vi "MoveBySteps.vi"(0 "Jiaxin_Stepper_Controller in":refnum<class "Jiaxin_Stepper_Controller.lvclass">, 1 "Direction":enum16{"Forward", "Backwards"}(ring)=enum."Backwards", 5 "Steps":dbl, 7 "Channel":u16(ring)=1 items=["Channel1"=1, "Channel2"=2, "Channel3"=3, "Channel4"=4], 9 "Speed":u32, 11 "error in (no error)":errorcluster, 13 "Polarity":enum16{"Positive", "Negative"}(ring)) -> (4 "Jiaxin_Stepper_Controller out":refnum<class "Jiaxin_Stepper_Controller.lvclass">, 15 "error out":errorcluster)   [LabVIEW 2023, in "Jiaxin_Stepper_Controller.lvlib" / "Jiaxin_Stepper_Controller.lvclass"]
uses:
  Jiaxin_Stepper_Controller.lvclass
  Jiaxin_Stepper_Controller.lvclass/Jiaxin_Stepper_Controller.ctl
  Interfaces/AbstractInstrumentClasses/TranslationStages_LV/TranslationStagesComm Messages/StageMoveDone Msg/StageMoveDone Msg.lvclass
  <vilib>/ActorFramework/Actor/Actor.lvclass
  UIs/TranslationStage_UI/TranslationStage_UI/StageMoveDone_For_UI.ctl
  typedefs/typedefs.lvlib
  C:/Program Files/National Instruments/LabVIEW 2023/vi.lib/ActorFramework/Actor/Actor.lvclass
  C:/Users/quantum/Documents/LVDAQ/ConcreteClasses/ConcreteInstrumentClasses/Jiaxin_Stepper_Controller/Jiaxin_Stepper_Controller/Jiaxin_Stepper_Controller.lvclass
  C:/Users/quantum/Documents/LVDAQ/Interfaces/InitDeinitInterface/InitDeinit/InitDeinit.lvclass
  C:/Users/quantum/Documents/LVDAQ/Interfaces/AbstractInstrumentClasses/TranslationStages_LV/TranslationStageInterface/TranslationStagesInterface.lvclass
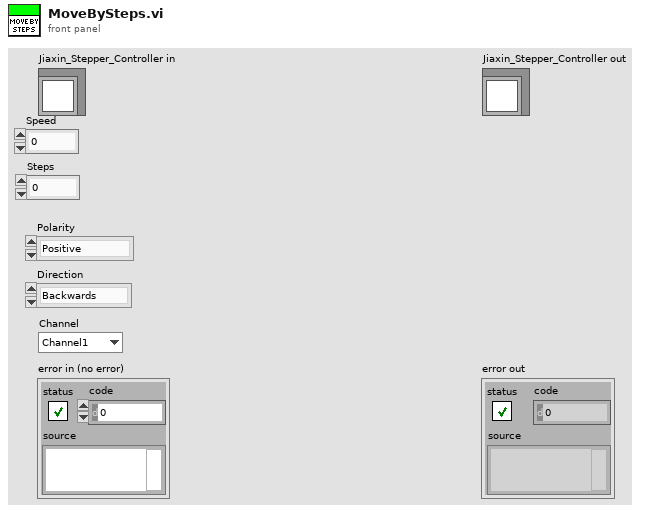
[diagram p1: front panel]
types:
  T1 = typedef "typedefs.lvlib/StageMoveDone_For_UI.ctl" = cluster{"CH1 Pos":dbl, "CH2 Pos":dbl, "CH3 Pos":dbl, "CH4 Pos":dbl, "Home?":bool}
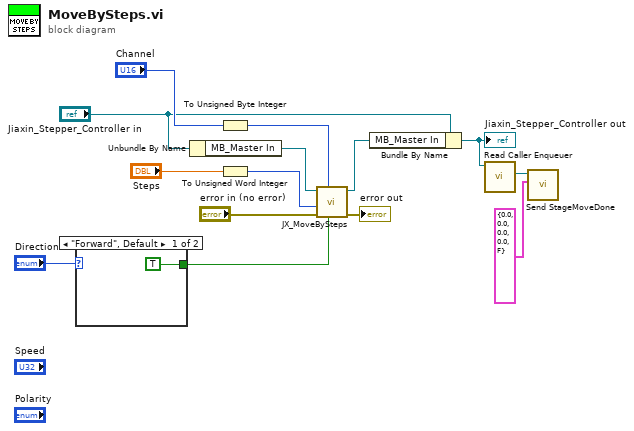
[diagram p0: block diagram]
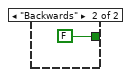
[diagram p2: hidden frame]
diagram:
  n1 = case shown="\"Forward\", Default" "Direction" {
    tunnel: [TRUE ("Direction") FALSE ("Direction")] -> w11
    frame "Forward", Default {
    }
    frame "Backwards" {
    }
  }
  n2 = Unbundle By Name("Jiaxin_Stepper_Controller in") -> ("MB_Master In"=w6:refnum<class "MB_Master.lvclass">)
  n3 = To Unsigned Byte Integer(number="Channel") -> (unsigned 8bit integer=w9:u8)
  n4 = To Unsigned Word Integer(number="Steps") -> (unsigned 16bit integer=w7:u16)
  n5 = call "JX_MoveBySteps.vi"("Direction"=w11, "Channel"=w9, "error in (no error)"="error in (no error)", "Steps"=w7, "Jiaxin_Stepper_Controller.lvlib:MB Serial Master:MB_Master"=w6) -> ("error out"=→"error out":errorcluster, "Jiaxin_Stepper_Controller.lvlib:MB Serial Master:MB_Master"=w5:refnum<class "MB_Master.lvclass">)  [unwired: 5 in]
  n6 = Bundle By Name(cluster="Jiaxin_Stepper_Controller in", "MB_Master In"=w5) -> (w2:refnum<class "Jiaxin_Stepper_Controller.lvclass">)
  "Jiaxin_Stepper_Controller out" <- w2
  n7 = call <vilib>:"Read Caller Enqueuer.vi"("Actor"=w2) -> ("Caller Enqueuer"=w3:refnum<class "Message Enqueuer.lvclass">)  [unwired: 10 in]
  n8 = call "Send StageMoveDone.vi"("Positions"=T1 {"CH1 Pos"=0.0, "CH2 Pos"=0.0, "CH3 Pos"=0.0, "CH4 Pos"=0.0, "Home?"=FALSE}, "Message Enqueuer"=w3) -> ()  [unwired: 8 in, 2 out]
